vi "TTL_check.vi"(8 "error in (no error)":errorcluster, 11 "TTL_input in":refnum<class "TTL_input.lvclass">) -> (0 "error out":errorcluster, 3 "TTL_input out":refnum<class "TTL_input.lvclass">)   [LabVIEW 2013, in "TTL_input.lvclass"]
uses:
  TTL_input.lvclass
  TTL_input.lvclass/TTL_input.ctl
  <vilib>/DAQmx/read.llb/DAQmx Read (Digital 1D Bool 1Chan 1Samp).vi
  Globals.vi
  <vilib>/DAQmx/miscellaneous.llb/DAQmx Fill In Error Info.vi
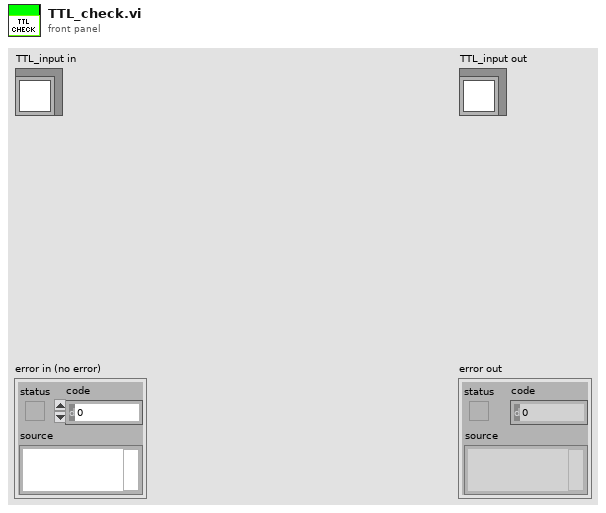
[diagram p1: front panel]
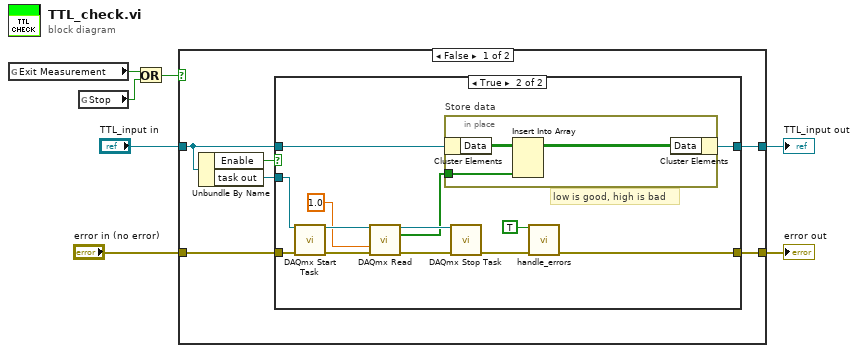
[diagram p0: block diagram]
diagram:
  n1 = global read "Globals.vi" "Exit Measurement"() -> (w4:bool)
  n2 = global read "Globals.vi" "Stop"() -> (w3:bool)
  n3 = Or(x=w4, y=w3) -> (x .or. y?=w2:bool)
  n4 = case shown="False" w2 {
    tunnel: [w13 w32] -> w5
    tunnel: [w9 w33] -> w6
    tunnel: "TTL_input in" -> [w10 w33]
    tunnel: "error in (no error)" -> [w8 w32]
    frame False {
      n5 = Unbundle By Name(w10) -> ("Enable"=w12:bool, "task out"=w11:refnum<k21>)
      n6 = case shown="True" w12 {
        tunnel: w8 -> [w15 w28]
        tunnel: [w15 w22] -> w13
        tunnel: w11 -> [_ w21]
        tunnel: w10 -> [w14 w20]
        tunnel: [w14 w18] -> w9
        frame False {
        }
        frame True {
          # "low is good, high is bad"
          n7 = call <vilib>:"DAQmx Start Task.vi"("task/channels in"=w21, "error in"=w28) -> ("task out"=w26:refnum<k21>, "error out"=w27:errorcluster)  [unwired: 12 in]
          n8 = call-poly <vilib>:"DAQmx Read.vi"("task/channels in"=w26, "timeout"=1.0, "error in"=w27) -> ("task out"=w24:refnum<k21>, "data"=w19:bool[], "error out"=w17:errorcluster)  [unwired: 10 in]
          n9 = in-place "Store data" {
            in-place-border: w19 -> [w30]
            n10 = in-place-cluster #1(w20) -> ("Data"=w31:bool[][])
            n11 = Insert Into Array(array=w31, new element=w30) -> (w29:bool[][])  [unwired: 2 in]
            n12 = in-place-cluster #1("Data"=w29) -> (w18:refnum<class "TTL_input.lvclass">)
          }
          n13 = call <vilib>:"DAQmx Stop Task.vi"("task/channels in"=w24, "error in"=w17) -> ("error out"=w23:errorcluster)  [unwired: 12 in, 1 out]
          n14 = call "handle_errors.vi"("Exit Operation"=TRUE ("Exit Measurement"), "error in (no error)"=w23) -> ("error out"=w22:errorcluster)  [unwired: 13 in]
        }
      }
    }
    frame True {
    }
  }
  "error out" <- w5
  "TTL_input out" <- w6
